vi "FTW-Actor-Initialize.vi"(0 "FTW Actor Instance Type":refnum<class "FTW-ScripterStep-Base.lvclass">, 5 "Initialization Job Sequence":string, 7 "Actor Instance Configuration":string, 11 "error in":errorcluster) -> (4 "FTW Actor Instance":refnum<class "FTW-ScripterStep-Base.lvclass">, 6 "Incoming Requests":refnum<event-registration>, 8 "Local Messages":refnum<event-registration>, 15 "error out":errorcluster)   [LabVIEW 2015, in "FTW-ScripterStep-Base.lvclass"]
uses:
  FTW-ScripterStep-Base.lvclass
  source/actor/Message/Request/FTW-Message-IncomingRequest.lvclass
  source/actor/Message/Base/FTW-Message.lvclass
  source/actor/Instance/FTW-ActorInstance.lvclass
panel:
  # "Inputs"
  # "Outputs"
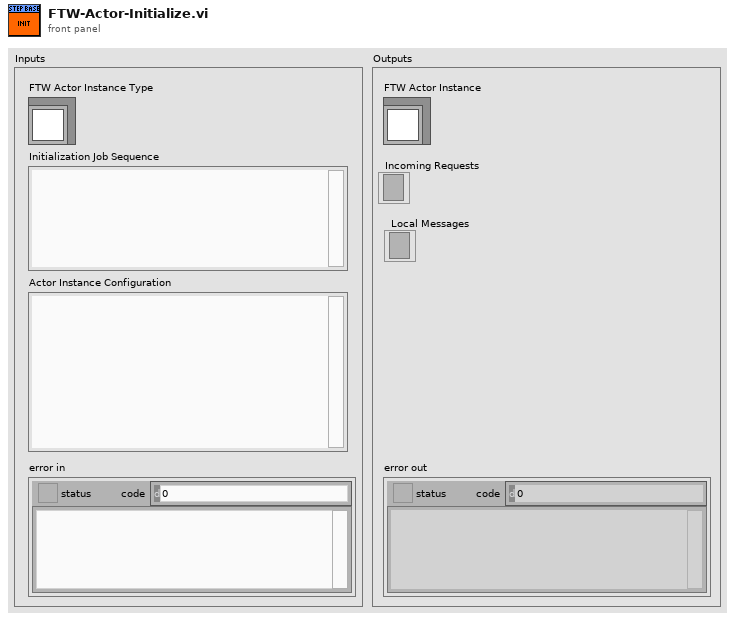
[diagram p1: front panel]
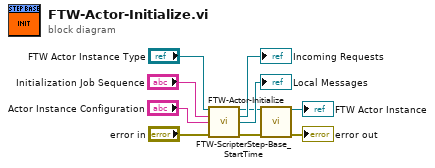
[diagram p0: block diagram]
diagram:
  n1 = call-parent "FTW-Actor-Initialize.vi"("FTW Actor Instance Type"="FTW Actor Instance Type", "Initialization Job Sequence"="Initialization Job Sequence", "Actor Instance Configuration"="Actor Instance Configuration", "error in"="error in") -> ("FTW Actor Instance"=w3:refnum<class "FTW-ScripterStep-Base.lvclass">, "Incoming Requests"=→"Incoming Requests":refnum<event-registration>, "Local Messages"=→"Local Messages":refnum<event-registration>, "error out"=w4:errorcluster)  [unwired: 8 in]
  n2 = call-dynamic "FTW-ScripterStep-Base_StartTime.vi"("FTW-ScripterStep-Base in"=w3, "error in (no error)"=w4) -> ("FTW-ScripterStep-Base out"=→"FTW Actor Instance":refnum<class "FTW-ScripterStep-Base.lvclass">, "error out"=→"error out":errorcluster)  [unwired: 12 in]
